vi "AE_AllStages_Action_ByRef.vi"(6 "Velocity":dbl, 7 "Abort":refnum<vi>, 8 "Positions":dbl[](array[numeric]), 9 "Axis":bool[](array[boolean]), 10 "Stage ID":string, 11 "Action":T1=enum."MVR") -> (0 "Position Out":dbl[](array[numeric]), 1 "Status":bool, 2 "Special Function Out":string, 5 "Valid handle":bool)   [LabVIEW 2014]
uses:
  Controls/StageStates.ctl
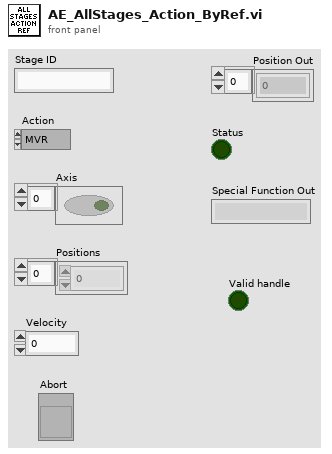
[diagram p1: front panel]
types:
  T1 = typedef "StageStates.ctl" = enum16{"POSITION", "MVR", "MOVE", "HALT", "ONTARGET", "ERROR", "EXIT", "HOME", "ZEROPOS", "NANOPOS", "QUIT", "ANALOG"}
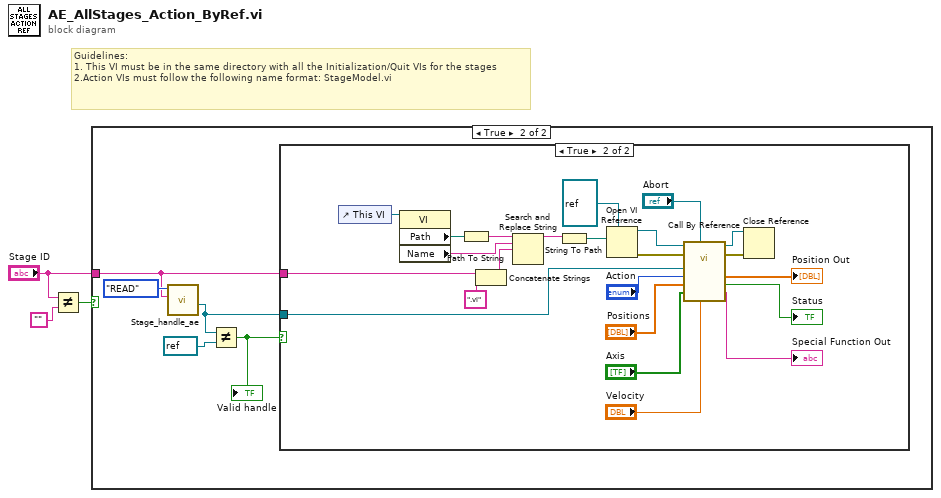
[diagram p0: block diagram]
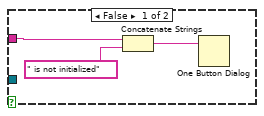
[diagram p3: hidden frame]
diagram:
  # "Guidelines:\n1. This VI must be in the same directory with all the Initialization/Quit VIs for the stages\n2.Action VIs must follow the following name format: StageModel.vi"
  n1 = Not Equal?(x="Stage ID", y="") -> (x != y?=w1:bool)
  n2 = case shown="True" w1 {
    tunnel: "Stage ID" -> [_ w4]
    frame False {
    }
    frame True {
      n3 = call "Stage_handle_ae.vi"("StageID"=w4, "Enum"=enum16{"WRITE", "READ"}."READ") -> ("Visa Out"=w5:refnum<visa-resource-name>)  [unwired: 9 in]
      n4 = Not Equal?(x=w5, y=refnum<visa-resource-name> refnum ("Visa Out")) -> (x != y?=w6:bool)
      "Valid handle" <- w6
      n5 = case shown="True" w6 {
        tunnel: w4 -> [w11 w30]
        tunnel: w5 -> [_ w18]
        frame False {
          n6 = Concatenate Strings(w11, " is not initialized" ("string")) -> (w9:string)
          n7 = One Button Dialog(message=w9) -> ()  [unwired: 1 in, 1 out]
        }
        frame True {
          n8 = control-ref of="This VI"() -> (w34:refnum<vi>)
          n9 = property class="VI"(reference=w34) -> ("Path"=w33:path, "Name"=w31:string)  [unwired: 1 in, 2 out]
          n10 = Path To String(path=w33) -> (string=w32:string)
          n11 = Concatenate Strings(w30, ".vi" ("string")) -> (w23:string)
          n12 = Search and Replace String(input string=w32, search string=w31, replace string=w23) -> (result string=w29:string)  [unwired: 5 in, 3 out]
          n13 = String To Path(string=w29) -> (path=w28:path)
          n14 = Open VI Reference(type specifier VI Refnum (for type only)=refnum<vi> refnum, vi path=w28) -> (vi reference=w16:refnum<vi>, error out=w25:errorcluster)  [unwired: 4 in]
          n15 = call-by-ref "?"(reference=w16, error in=w25, "Velocity"="Velocity", "Abort"="Abort", "Axis"="Axis", "Positions In"="Positions", "Action"="Action", "VISA In"=w18) -> (reference out=w26:refnum<vi>, error out=w24:errorcluster, "Special Function Out"=→"Special Function Out":string, "Status"=→"Status":bool, "Position Out"=→"Position Out":dbl[])  [unwired: 2 in, 1 out]
          n16 = Close Reference(reference=w26, error in (no error)=w24) -> ()  [unwired: 1 out]
        }
      }
    }
  }
